vi "DrumSeq_Continuous_Example.vi"() -> ()   [LabVIEW 2019]
uses:
  <vilib>/Rock Robotics/WPI/ThirdParty/JAS_Junk/TrajLib/Enum/AutoHelperSequence_Step_Enum.ctl
  <vilib>/Rock Robotics/WPI/ThirdParty/JAS_Junk/TrajLib/VI/Util_GetTime_U32.vi
  <vilib>/Rock Robotics/WPI/ThirdParty/JAS_Junk/TrajLib/VI/BoolCmd_Recv_Internal.vi
  <vilib>/Rock Robotics/WPI/ThirdParty/JAS_Junk/TrajLib/Timer_New.vi
  <vilib>/Rock Robotics/WPI/ThirdParty/JAS_Junk/TrajLib/VI/BoolCmd_Send_Internal.vi
  <vilib>/Rock Robotics/WPI/ThirdParty/JAS_Junk/TrajLib/VI/BoolCmd_ObtainQueue.vi
  <vilib>/Rock Robotics/WPI/ThirdParty/JAS_Junk/TrajLib/VI/Util_GetTime_U64.vi
  <vilib>/Utility/semaphor.llb/Obtain Semaphore Reference.vi
  <vilib>/Rock Robotics/WPI/ThirdParty/JAS_Junk/TrajLib/Timer_Reset.vi
  <vilib>/Rock Robotics/WPI/ThirdParty/JAS_Junk/TrajLib/VI/Timer_Restart.vi
  <vilib>/Rock Robotics/WPI/ThirdParty/JAS_Junk/TrajLib/Timer_HasPeriodPassedOnce.vi
  <vilib>/Rock Robotics/WPI/ThirdParty/JAS_Junk/TrajLib/Trajectory_Library.lvlib
panel:
  out "Speed Demand":dbl
  in  "Teleop Action\nCancel":bool
  out "Auto Step Number":T1
  out "Auto\nActive":bool
  in  "Start\nAutonomous":bool
  in  "Teleop Action\nCapture":bool
  out "Hand Control \nOutput":bool
  out "Waveform Chart":cluster{dbl, i16, i16}(graph)
  out "Arm Control\nOutput":bool
  # "CONTINUOUS DRUM SEQUENCER"
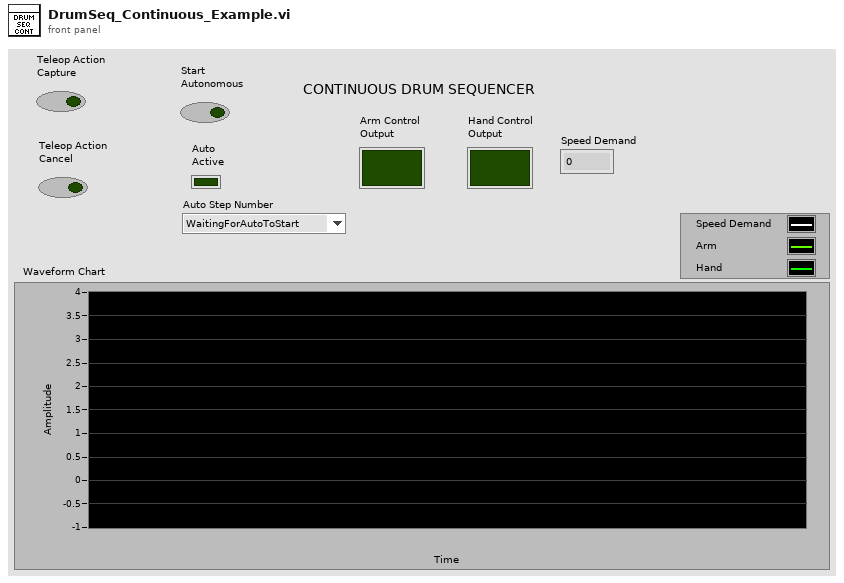
[diagram p1: front panel]
types:
  T1 = typedef "Trajectory_Library.lvlib/AutoHelperSequence_Step_Enum.ctl" = enum16{"WaitingForAutoToStart", "Step 1", "Step 2", "Step 3", "Step 4", "Step 5", "Step 6", "Step 7", "Step 8", "Step 9", "Step 10", "Step 11", "Step 12", "Step 13", "Step 14", "Step 15", "Step 16", "Step 17", "Step 18", "Step 19", "Step 20", "Step 21", "Step 22", "Step 23", "Step 24", "Step 25", "Step 26", "Step 27", "Step 28", "Step 29", "Step 30", "Step 31", "Step 32", "AutoDone"}
  T2 = typedef "Trajectory_Library.lvlib/DrumSequence_Step_Enum.ctl" = enum16{"Do Nothing", "Step 1", "Step 2", "Step 3", "Step 4", "Step 5", "Step 6", "Step 7", "Step 8", "Step 9", "Step 10", "Step 11", "Step 12", "Step 13", "Step 14", "Step 15", "Step 16", "Step 17", "Step 18", "Step 19", "Step 20", "Step 21", "Step 22", "Step 23", "Step 24", "Step 25", "Step 26", "Step 27", "Step 28", "Step 29", "Step 30", "Step 31", "Step 32", "Cancel", "Initialize", "Error"}
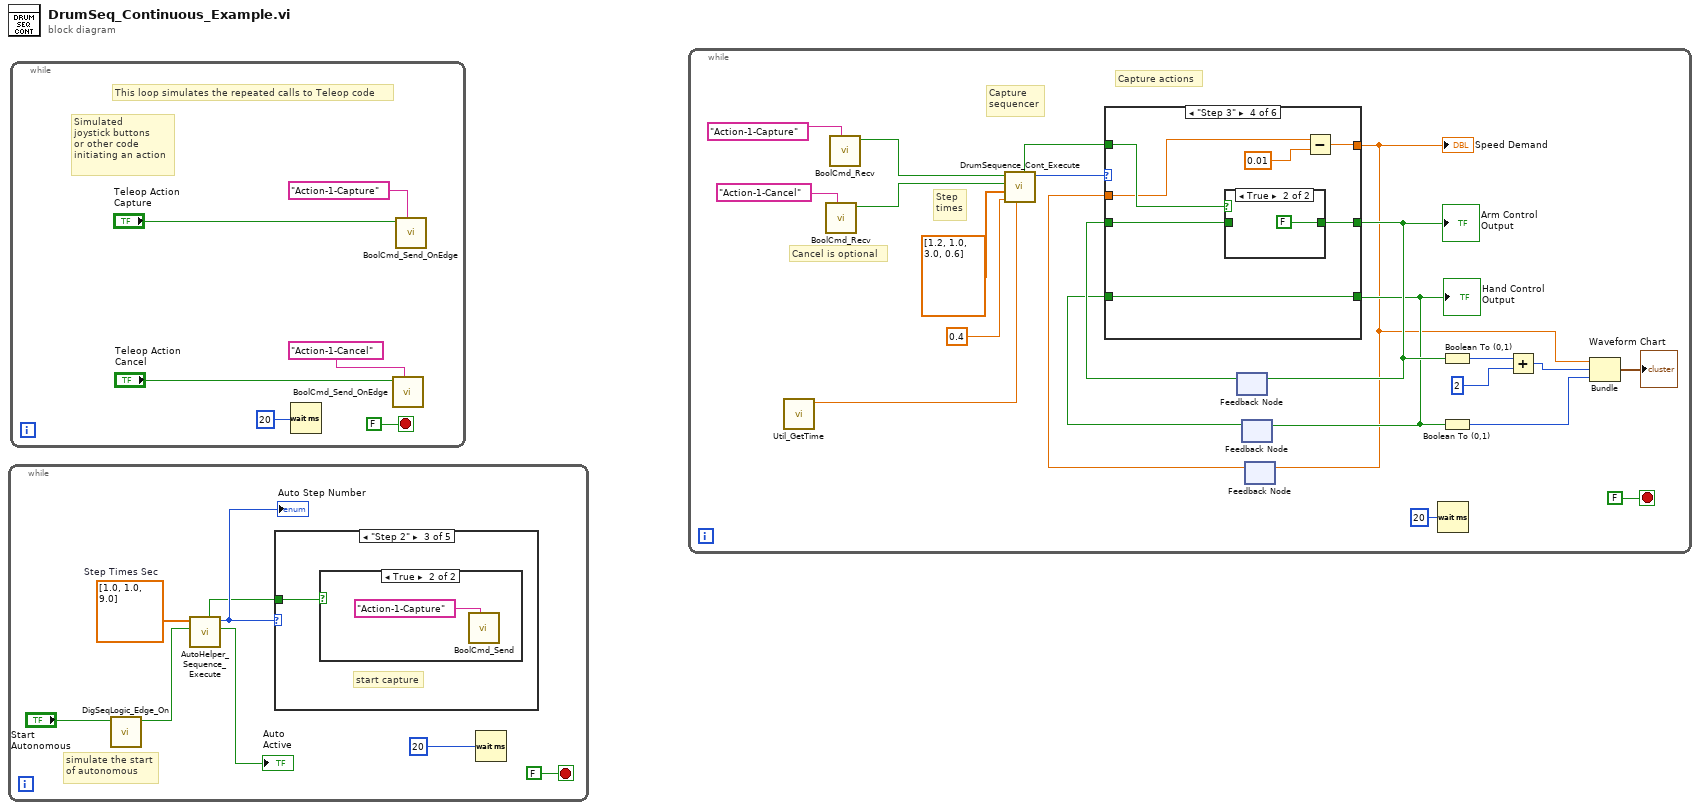
[diagram p0: block diagram]
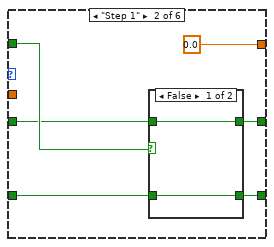
[diagram p3: hidden frame]
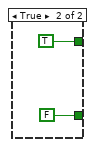
[diagram p4: hidden frame]
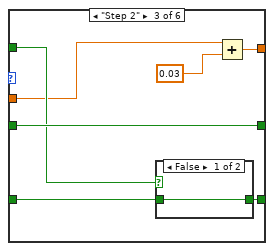
[diagram p5: hidden frame]
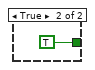
[diagram p6: hidden frame]
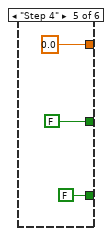
[diagram p8: hidden frame]
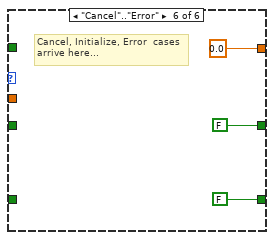
[diagram p9: hidden frame]
diagram:
  n1 = while {
    stop <- FALSE stop-if-true
    w5 = dbl[] [1.0, 1.0, 9.0]  # Step Times Sec
    # "simulate the start\nof autonomous"
    n2 = call <vilib>:"DigSeqLogic_Edge_On.vi"("Input"="Start\nAutonomous") -> ("On Edge"=w4:bool)  [unwired: 10 in]
    n3 = call <vilib>:"AutoHelper_Sequence_Execute.vi"("Initiate"=w4, "Step Times Sec"=w5) -> ("Seq  Active"=→"Auto\nActive":bool, "Step Number State"=w3:T1, "New Step"=w2:bool)  [unwired: 5 in, 2 out]
    "Auto Step Number" <- w3
    n4 = case shown="\"Step 2\"" w3 {
      tunnel: w2 -> [_ _ w9 _ _]
      frame "WaitingForAutoToStart", Default {
        # "do nothing"
      }
      frame "Step 1" {
        # "do nothing"
      }
      frame "Step 2" {
        # "start capture"
        n5 = case shown="True" w9 {
          frame False {
          }
          frame True {
            n6 = call <vilib>:"BoolCmd_Send.vi"("Command Name"="Action-1-Capture") -> ()  [unwired: 10 in, 1 out]
          }
        }
      }
      frame "Step 3" {
        # "Do nothing"
      }
      frame "AutoDone" {
        # "Auto is done."
      }
    }
    n7 = Wait (ms)(milliseconds to wait=u32 20 ("milliseconds to wait 2")) -> ()  [unwired: 1 out]
  }
  n8 = while {
    stop <- FALSE stop-if-true
    # "Simulated\njoystick buttons\nor other code \ninitiating an action"
    # "This loop simulates the repeated calls to Teleop code"
    n9 = Wait (ms)(milliseconds to wait=u32 20) -> ()  [unwired: 1 out]
    n10 = call <vilib>:"BoolCmd_Send_OnEdge.vi"("Command Name"="Action-1-Cancel", "Value"="Teleop Action\nCancel") -> ()  [unwired: 9 in, 1 out]
    n11 = call <vilib>:"BoolCmd_Send_OnEdge.vi"("Command Name"="Action-1-Capture", "Value"="Teleop Action\nCapture") -> ()  [unwired: 9 in, 1 out]
  }
  n12 = while {
    stop <- FALSE stop-if-true
    # "Step\ntimes"
    # "Cancel is optional"
    # "Capture actions"
    # "Capture\nsequencer"
    n13 = call <vilib>:"Util_GetTime.vi"() -> ("FPGA_Time_Seconds"=w30:dbl)  [unwired: 9 in, 2 out]
    n14 = call <vilib>:"BoolCmd_Recv.vi"("Command Name"="Action-1-Cancel") -> ("New Request"=w20:bool)  [unwired: 9 in, 1 out]
    n15 = call <vilib>:"BoolCmd_Recv.vi"("Command Name"="Action-1-Capture") -> ("New Request"=w21:bool)  [unwired: 9 in, 1 out]
    n16 = call <vilib>:"DrumSequence_Cont_Execute.vi"("Pass_Through_Time"=w30, "Cancel Time Sec"=0.4, "Step Times Sec"=dbl[] [1.2, 1.0, 3.0, 0.6], "Cancel"=w20, "Initiate"=w21) -> ("Step Number State"=w33:T2, "New Step"=w19:bool)  [unwired: 2 in, 3 out]
    n17 = feedback #1() -> (w32:bool)  [unwired: 1 in]
    n18 = feedback #2() -> (w31:bool)  [unwired: 1 in]
    n19 = feedback #3() -> (w18:dbl)  [unwired: 1 in]
    n20 = case shown="\"Step 3\"" w33 {
      tunnel: [w41 w47 w57 w67 FALSE FALSE] -> w23
      tunnel: [w40 w46 w58 w66 FALSE FALSE] -> w22
      tunnel: w32 -> [w41 w44 w57 w64 _ _]
      tunnel: w31 -> [w40 w43 w55 w66 _ _]
      tunnel: w19 -> [_ w45 w56 w65 _ _]
      tunnel: [w39 0.0 w54 w63 0.0 0.0] -> w17
      tunnel: w18 -> [w39 _ w53 w62 _ _]
      frame "Do Nothing", Default {
      }
      frame "Step 1" {
        n21 = case shown="False" w45 {
          tunnel: [w49 TRUE] -> w47
          tunnel: [w48 FALSE] -> w46
          tunnel: w44 -> [w49 _]
          tunnel: w43 -> [w48 _]
          frame False {
          }
          frame True {
          }
        }
      }
      frame "Step 2" {
        n22 = case shown="False" w56 {
          tunnel: [w59 TRUE] -> w58
          tunnel: w55 -> [w59 _]
          frame False {
          }
          frame True {
          }
        }
        n23 = Add(x=w53, y=0.03) -> (x+y=w54:dbl)
      }
      frame "Step 3" {
        n24 = case shown="True" w65 {
          tunnel: [w68 FALSE] -> w67
          tunnel: w64 -> [w68 _]
          frame False {
          }
          frame True {
          }
        }
        n25 = Subtract(x=w62, y=0.01) -> (x-y=w63:dbl)
      }
      frame "Step 4" {
      }
      frame "Cancel".."Error" {
        # "Cancel, Initialize, Error  cases\narrive here..."
      }
    }
    "Arm Control\nOutput" <- w23
    "Hand Control \nOutput" <- w22
    "Speed Demand" <- w17
    n26 = feedback-in #1(w23) -> ()
    n27 = feedback-in #2(w22) -> ()
    n28 = feedback-in #3(w17) -> ()
    n29 = Wait (ms)(milliseconds to wait=u32 20) -> ()  [unwired: 1 out]
    n30 = Boolean To (0,1)(Boolean=w23) -> (0, 1=w27:i16)
    n31 = Boolean To (0,1)(Boolean=w22) -> (0, 1=w25:i16)
    n32 = Add(x=w27, y=i16 2) -> (x+y=w26:i16)
    n33 = Bundle(w17, w26, w25) -> (→"Waveform Chart":cluster{dbl, i16, i16})  [unwired: 1 in]
  }
